vi "Read Power.vi"(0 "SG Path Power Meter Accessor in":refnum<class "SG 2250 Path Accessor.lvclass">, 5 "Cal point in":T1, 11 "error in (no error)":errorcluster) -> (4 "SG Path Power Meter Accessor out":refnum<class "SG 2250 Path Accessor.lvclass">, 6 "Power (dBm)":dbl, 15 "error out":errorcluster)   [LabVIEW 2023, in "NI-568x RF Power Meter.lvlib" / "SG 2250 Path Accessor.lvclass"]
uses:
  SG 2250 Path Accessor.lvclass
  Public/Base Classes/Scalar/Scalar Path/Type Definitions/Cal Point.ctl
  Power Meter/Power Meter.lvclass
  Power Meter/Power Meter.lvclass/Power Meter.ctl
  Power Meter/Properties/Read Resource Name.vi
  Instruments/Power Meter/Power Meter Factory/Power Meter Factory.lvclass
  Public/Base Classes/Scalar/Scalar Path/Scalar Path.lvclass
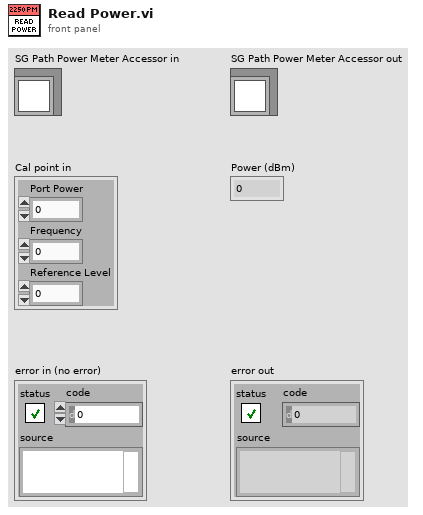
[diagram p1: front panel]
types:
  T1 = typedef "RFFixtureCharact.Public.lvlib/Scalar Path.lvclass/Cal Point.ctl" = cluster{"Port Power":dbl, "Frequency":dbl, "Reference Level":dbl}
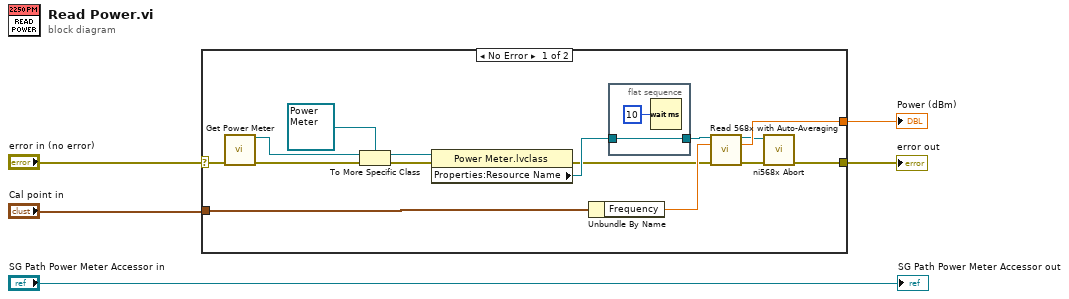
[diagram p0: block diagram]
diagram:
  n1 = case shown="No Error" "error in (no error)" {
    selector: "error in (no error)" -> [w15 w23]
    tunnel: [w19 w23] -> w5
    tunnel: [w20 _] -> w4
    tunnel: "Cal point in" -> [w9 _]
    frame No Error {
      n2 = call "Get Power Meter.vi"("error in (no error)"=w15) -> ("Power Meter Base out"=w16:refnum<class "Power Meter Base.lvclass">, "error out"=w17:errorcluster)  [unwired: 13 in]
      n3 = To More Specific Class(target class=refnum<class "Power Meter.lvclass"> refnum ("PM NI568X in"), reference=w16, error in=w17) -> (specific class reference=w13:refnum<class "Power Meter.lvclass">, error out=w14:errorcluster)
      n4 = property class="Power Meter.lvclass"(reference=w13, error in=w14) -> (error out=w6:errorcluster, "Properties:Resource Name"=w7:refnum<k15>)  [unwired: 1 out]
      n5 = Unbundle By Name(w9) -> ("Frequency"=w12:dbl)
      n6 = flat-sequence {
        tunnel: [w21] -> w8
        tunnel: w7 -> [w21]
        frame #0 {
          n7 = Wait (ms)(milliseconds to wait=u32 10) -> ()  [unwired: 1 out]
        }
      }
      n8 = call "Read 568x with Auto-Averaging.vi"("reference"=w8, "Frequency (Hz)"=w12, "error in (no error)"=w6) -> ("reference out"=w10:refnum<k15>, "measurement"=w20:dbl, "error out"=w11:errorcluster)  [unwired: 10 in]
      n9 = call <instrlib>:"ni568x Abort.vi"("error in"=w11, "instrument handle"=w10) -> ("error out"=w19:errorcluster)  [unwired: 8 in, 1 out]
    }
    frame Error {
    }
  }
  "error out" <- w5
  "Power (dBm)" <- w4
  "SG Path Power Meter Accessor out" <- "SG Path Power Meter Accessor in"
